vi "Newport Powermeter Control Program(ver0.1).vi"() -> ()   [LabVIEW 2018]
panel:
  in  "stop":bool
  in  "Timer(sec)":dbl
  out "Power Meter":cluster{"Power Value":dbl[], "Time":dbl[]}(graph)
  out "Device Name":string
  out "Optical  Power":string[](array[string])
  out "Calibrated Time":dbl=1000.0
  in  "Sample per second":dbl=1.0
  out "Time":dbl[](array[numeric])
  out "Power Value":dbl[](array[numeric])
  # "Real-Time Optical Power Measurement Program"
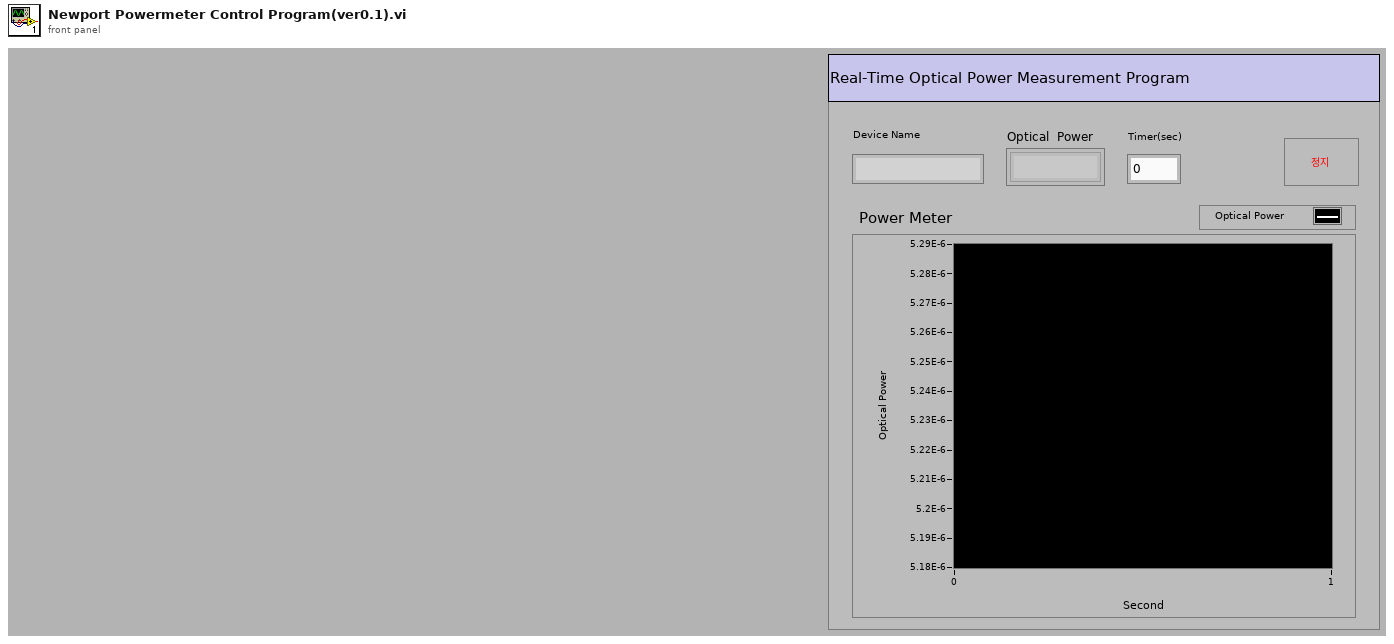
[diagram p1: front panel]
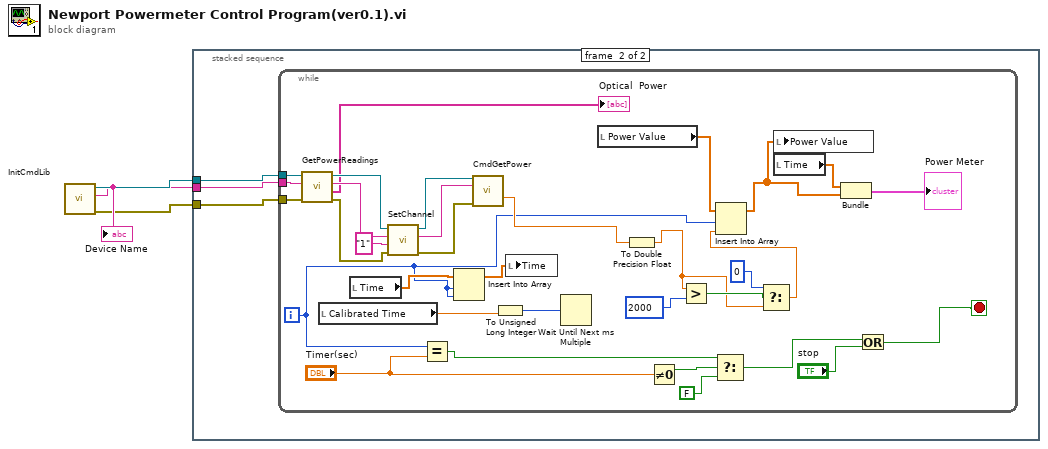
[diagram p0: block diagram]
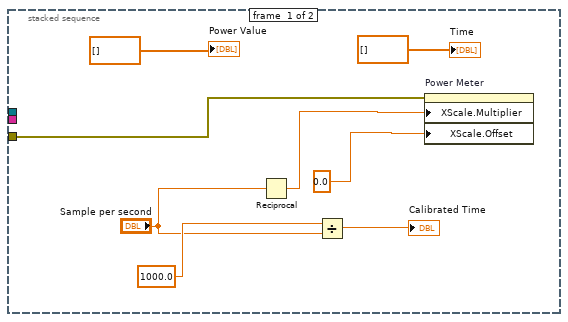
[diagram p2: hidden frame]
diagram:
  n1 = call "InitCmdLib.vi"() -> ("error out"=w1:errorcluster, "Device Key"=w2:string, "CmdLib"=w3:refnum<k24>)  [unwired: 9 in]
  "Device Name" <- w2
  n2 = stacked-sequence {
    tunnel: w3 -> [_ w14]
    tunnel: w2 -> [_ w13]
    tunnel: w1 -> [w4 w12]
    frame #0 {
      n3 = Reciprocal(x="Sample per second") -> (1/x=w6:dbl)
      n4 = Divide(x=1000.0, y="Sample per second") -> (x/y=→"Calibrated Time":dbl)
      n5 = property on="Power Meter" class="XYGraph (엄격한)"(error in=w4, "XScale.Multiplier"=w6, "XScale.Offset"=0.0) -> ()  [unwired: 1 in, 2 out]
      "Power Value" <- dbl[] []
      "Time" <- dbl[] []
    }
    frame #1 {
      n6 = while {
        tunnel: w14 -> [w46]
        tunnel: w13 -> [w45]
        tunnel: w12 -> [w44]
        i -> [w27]
        stop <- w25 stop-if-true
        n7 = call "GetPowerReadings.vi"("error in"=w44, "Device Key In"=w45, "PM Cmds In"=w46) -> ("error out"=w41:errorcluster, "Power Readings"=→"Optical  Power":string[], "Device Key Out"=w42:string, "PM Cmds Out"=w43:refnum<k24>)  [unwired: 1 in]
        n8 = local read "Calibrated Time"() -> (w35:dbl)
        n9 = local read "Time"() -> (w31:dbl[])
        n10 = call "SetChannel.vi"("error in"=w41, "Channel 1 or 2"="1" ("channel"), "Device Key In"=w42, "PM Cmds In"=w43) -> ("error out"=w38:errorcluster, "Device Key Out"=w39:string, "PM Cmds Out"=w40:refnum<k24>)  [unwired: 1 in]
        n11 = Equal?(x=w27, y="Timer(sec)") -> (x = y?=w16:bool)
        n12 = Insert Into Array(array=w31, index=w27, new element=w27) -> (w30:dbl[])
        n13 = call "CmdGetPower.vi"("PM Cmds In"=w40, "Device Key In"=w39, "error in"=w38) -> ("Power Value"=w34:sgl)  [unwired: 8 in, 4 out]
        n14 = To Unsigned Long Integer(number=w35) -> (unsigned 32bit integer=w36:u32)
        n15 = local write "Time"(w30) -> ()
        n16 = Wait Until Next ms Multiple(millisecond multiple=w36) -> ()  [unwired: 1 out]
        n17 = local read "Power Value"() -> (w33:dbl[])
        n18 = To Double Precision Float(number=w34) -> (double precision float=w20:dbl)
        n19 = Not Equal To 0?(x="Timer(sec)") -> (x != 0?=w18:bool)
        n20 = Greater?(x=w20, y=2000) -> (0:w23:bool)
        n21 = Select(t=w16, s=w18, f=FALSE) -> (s? t:f=w17:bool)
        n22 = Select(t=0, s=w23, f=w20) -> (s? t:f=w21:dbl)
        n23 = Insert Into Array(array=w33, index=w27, new element=w21) -> (w28:dbl[])
        n24 = local write "Power Value"(w28) -> ()
        n25 = local read "Time"() -> (w29:dbl[])
        n26 = Bundle("Time"=w29, "Power Value"=w28) -> (→"Power Meter":cluster{"Time":dbl[], "Power Value":dbl[]})  [unwired: 1 in]
        n27 = Or(x=w17, y="stop") -> (x .or. y?=w25:bool)
      }
    }
  }
